vi "Check_End_Position.vi"(4 "Model       Roll      Pitch       Yaw (deg)":sgl[](array[numeric]) format="%#.2f", 5 "Exclude Array":T1[](array[typedef])=[{"Sizes"=[{"Max"=15000.0, "Min"=0.0}, {"Max"=1000.0, "Min"=-1000.0}, {"Max"=300.0, "Min"=0.0}], "Name"="Roughness Elements", "Exclude Type"=enum."Allow only vertical moves"}, {"Sizes"=[{"Max"=17000.0, "Min"=16000.0}, {"Max"=200.0, "Min"=-200.0}, {"Max"=-50.0, "Min"=-250.0}], "Name"="B204", "Exclude Type"=enum."Exclude completely"}] {"Sizes"."Min" format="%#.1f"; "Sizes"."Max" format="%#.1f"}, 6 "Volume Name":string, 7 "Traverse Name":string, 8 "Entire Space":T2=[{"Max"=15001.0, "Min"=12000.0}, {"Max"=1000.0, "Min"=-1000.0}, {"Max"=700.0, "Min"=0.0}] {"Min" format="%#.1f"; "Max" format="%#.1f"}, 9 "Probe Volume":T2=[{"Max"=15.0, "Min"=-15.0}, {"Max"=250.0, "Min"=0.0}, {"Max"=15.0, "Min"=-15.0}] {"Min" format="%#.1f"; "Max" format="%#.1f"}, 10 "New Position":sgl[](array[numeric])=[0.0, 0.0, 0.0] format="%.2f", 11 "Current position":sgl[](array[numeric])=[0.0, 0.0, 0.0] format="%.2f") -> (0 "Error Comments":string)   [LabVIEW 2020]
uses:
  Box_size.ctl
  Exclude_cluster.ctl
  Exclusion_type.ctl
panel:
  out "Numeric":i32
  # "X                Y                   Z"
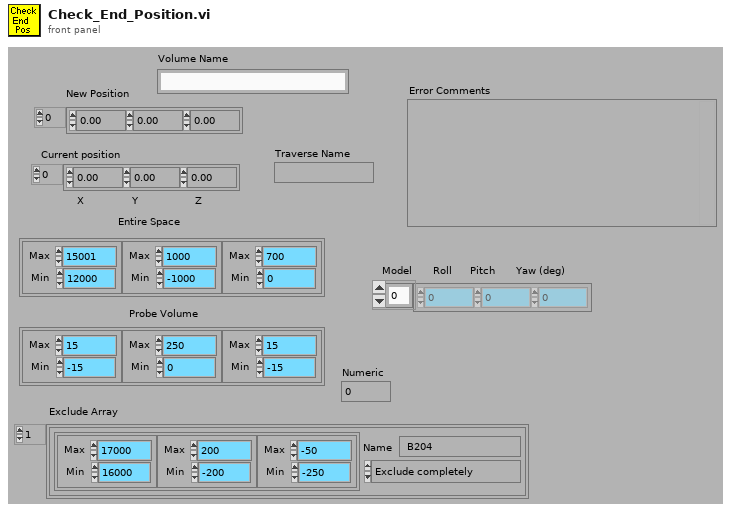
[diagram p1: front panel]
types:
  T1 = typedef "Exclude_cluster.ctl" = cluster{"Sizes":T2, "Name":string, "Exclude Type":T3}
  T2 = typedef "Box_size.ctl" = cluster{"Max":sgl, "Min":sgl}[]
  T3 = typedef "Exclusion_type.ctl" = enum16{"Exclude completely", "Allow only vertical moves"}
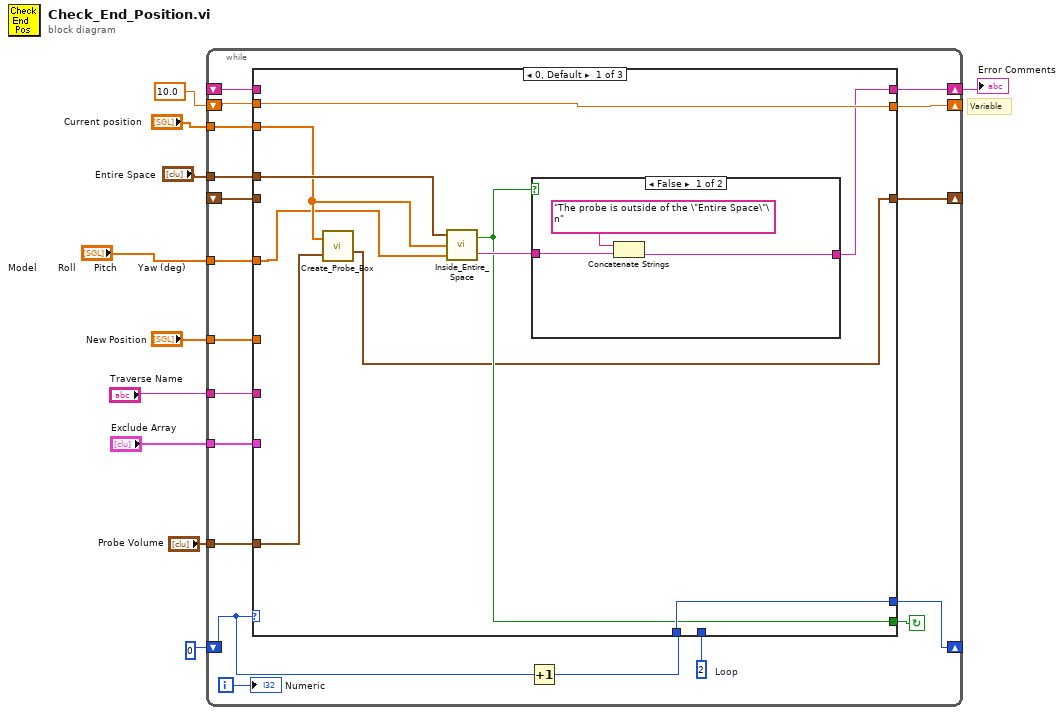
[diagram p0: block diagram]
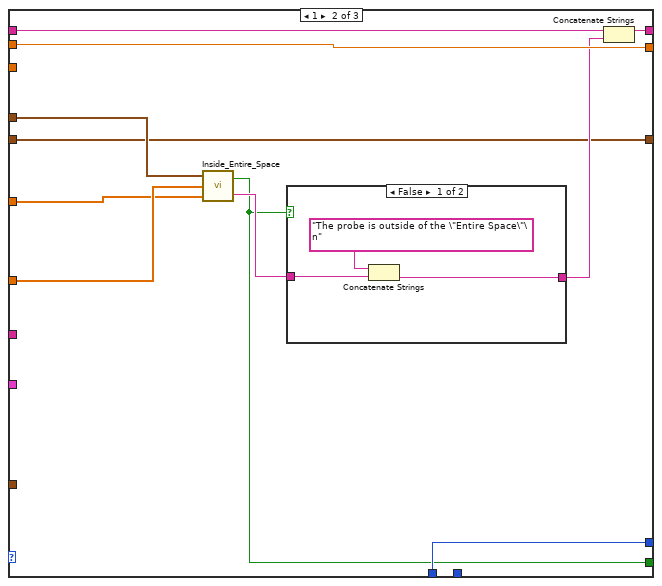
[diagram p3: hidden frame]
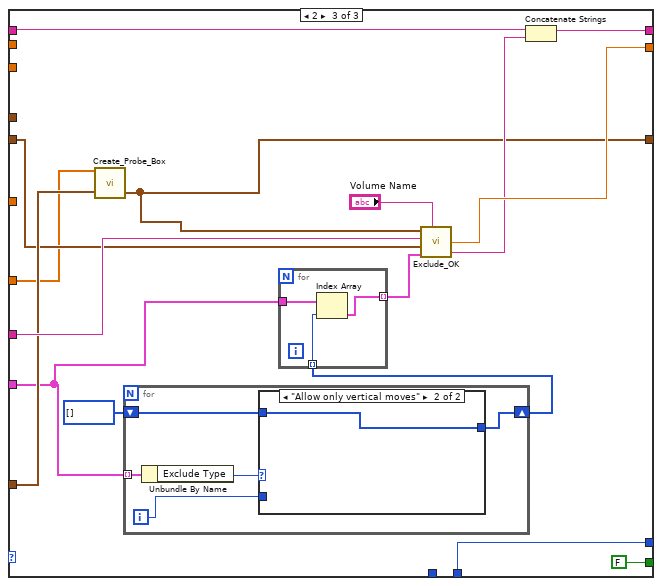
[diagram p5: hidden frame]
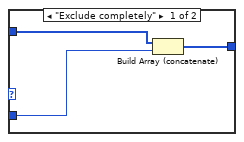
[diagram p6: hidden frame]
diagram:
  # "Variable"
  n1 = while {
    shift-left: _ -> [w13]
    shift-right: [w14] -> _
    tunnel: "Probe Volume" -> [w16]
    tunnel: "New Position" -> [w18]
    shift-left: _ -> [w19]
    shift-right: [w20] -> w6
    shift-left: 0 -> [w23]
    shift-right: [w22] -> _
    tunnel: "Traverse Name" -> [w24]
    tunnel: "Entire Space" -> [w25]
    tunnel: "Exclude Array" -> [w27]
    shift-left: 10.0 ("Separation Distance") -> [w29]
    shift-right: [w26] -> _
    tunnel: "Current position" -> [w12]
    tunnel: "Model       Roll      Pitch       Yaw (deg)" -> [w11]
    i -> [w15]
    stop <- w28 continue-if-true
    w17 = 2  # Loop
    n2 = Increment(x=w23) -> (x+1=w21:i32)
    n3 = case shown="0, Default" w23 {
      tunnel: w29 -> [w37 w52 _]
      tunnel: [w33 w47 FALSE ("Box Inside")] -> w28
      tunnel: w16 -> [w35 _ w69]
      tunnel: w27 -> [_ _ w61]
      tunnel: [w37 w52 w74] -> w26
      tunnel: w25 -> [w39 w54 _]
      tunnel: w24 -> [_ _ w73]
      tunnel: [w34 w48 w68] -> w22
      tunnel: w21 -> [w34 w48 _]
      tunnel: [w36 w50 w71] -> w20
      tunnel: w19 -> [_ w51 w72]
      tunnel: w18 -> [_ w45 w64]
      tunnel: w17 -> [_ _ w68]
      tunnel: [w31 w46 w67] -> w14
      tunnel: w13 -> [_ w46 w66]
      tunnel: w12 -> [w32 _ _]
      tunnel: w11 -> [w30 w44 _]
      frame 0, Default {
        n4 = call "Create_Probe_Box.vi"("Probe Volume"=w35, "Probe Position"=w32) -> ("Current Probe Volume"=w31:T2)
        n5 = call "Inside_Entire_Space.vi"("Model       Roll      Pitch       Yaw (deg)"=w30, "Current Position"=w32, "Envelope"=w39) -> ("Error Comments"=w38:string, "Box Inside"=w33:bool)  [unwired: 1 in]
        n6 = case shown="False" w33 {
          tunnel: w38 -> [w41 w43]
          tunnel: [w40 w43] -> w36
          frame False {
            n7 = Concatenate Strings("The probe is outside of the \"Entire Space\"\n" ("Format String"), w41) -> (w40:string)
          }
          frame True {
          }
        }
      }
      frame 1 {
        n8 = call "Inside_Entire_Space.vi"("Model       Roll      Pitch       Yaw (deg)"=w44, "Current Position"=w45, "Envelope"=w54) -> ("Error Comments"=w53:string, "Box Inside"=w47:bool)  [unwired: 1 in]
        n9 = case shown="False" w47 {
          tunnel: w53 -> [w56 w58]
          tunnel: [w55 w58] -> w49
          frame False {
            n10 = Concatenate Strings("The probe is outside of the \"Entire Space\"\n" ("Format String"), w56) -> (w55:string)
          }
          frame True {
          }
        }
        n11 = Concatenate Strings(w51, w49) -> (w50:string)
      }
      frame 2 {
        n12 = call "Create_Probe_Box.vi"("Probe Volume"=w69, "Probe Position"=w64) -> ("Current Probe Volume"=w67:T2)
        n13 = for {
          shift-right: [w79] -> w62
          shift-left: i32[] [] -> [w80]
          tunnel: w61 -> [w82] mode=indexing
          i -> [w78]
          n14 = Unbundle By Name(w82) -> ("Exclude Type"=w81:T3)
          n15 = case shown="\"Allow only vertical moves\"" w81 {
            tunnel: w80 -> [w85 w86]
            tunnel: [w84 w86] -> w79
            tunnel: w78 -> [w83 _]
            frame "Exclude completely" {
              n16 = Build Array (concatenate)(w85, w83) -> (w84:i32[])
            }
            frame "Allow only vertical moves" {
            }
          }
        }
        n17 = for {
          tunnel: w62 -> [w77] mode=indexing
          tunnel: w61 -> [w76]
          tunnel: [w75] -> w60 mode=indexing
          n18 = Index Array(array=w76, index=w77) -> (element=w75:T1)
        }
        n19 = call "Exclude_OK.vi"("Probe Volume"=w67, "Traverse Name"=w73, "Previous Probe Volume"=w66, "Exclude Array"=w60, "Volume Name"="Volume Name") -> ("Separation Distance"=w74:sgl, "Error Comments"=w70:string)  [unwired: 1 out]
        n20 = Concatenate Strings(w72, w70) -> (w71:string)
      }
    }
    "Numeric" <- w15
  }
  "Error Comments" <- w6
